vi "FGV_MacroCore.vi"(6 "Final Index":i32, 7 "MacroFGV_Commands":T1, 8 "Error In":errorcluster, 9 "Length":i32, 10 "Start Index":i32, 11 "Macro Command or Info (String)":string) -> (0 "Error Out":errorcluster, 1 "Info Table Array":string[](array[string]), 2 "File IO Cancelled/Error?":bool, 3 "Macro String Array":string[](array[string]), 5 "Saved Macro Path":path)   [LabVIEW 2012]
doc: "SciScan 1.2 160622\nThis is the main FGV which manages the Macro Data"
uses:
  FGV_MacroCore_Commands.ctl
  MacroFileIO_Commands.ctl
  FGV_Macro Settings to GFG_Command.ctl
  Macro Rule/subVIs/MacroRules_FGV_Commands.ctl
  Custom Controls/Setting File Types.ctl
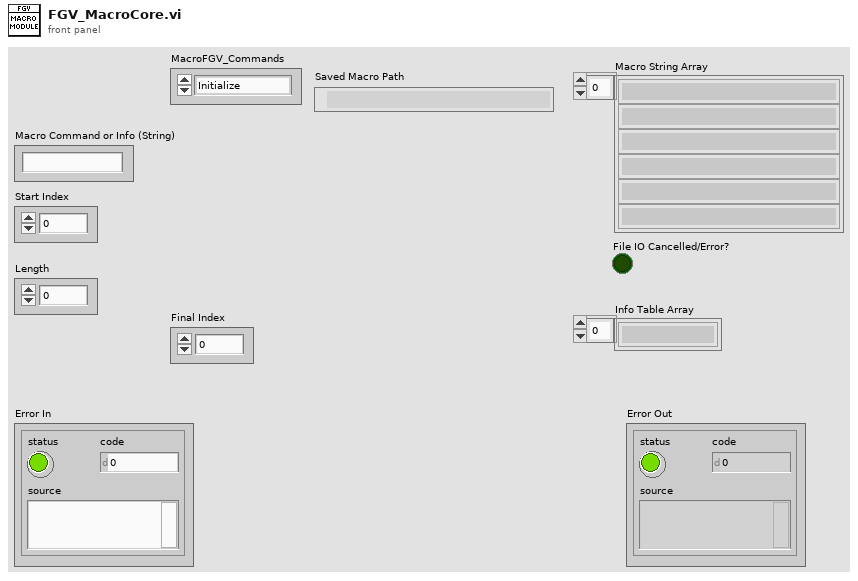
[diagram p1: front panel]
types:
  T1 = typedef "FGV_MacroCore_Commands.ctl" = enum16{"Initialize", "Get Array", "Load macro from file", "Insert Item", "Insert at End", "Edit Parameter String", "Delete instruction", "Move Items", "Save", "SaveAs", "UpdateInfoTable", "Edit Settings File", "New Macro", "Read Temp File", "Delete Multiple"}
  T2 = typedef "MacroFileIO_Commands.ctl" = enum16{"Get Macro Info", "Initialize", "New Macro", "Load Macro", "Save", "Save in today's folder", "Update Settings File", "Add Settings File", "Delete Settings File", "Update Macro Text", "Save As", "Read Temp File"}
  T3 = typedef "MacroRules_FGV_Commands.ctl" = enum16{"Read File", "Get All", "Get Param and Flags"}
  T4 = typedef "FGV_Macro Settings to GFG_Command.ctl" = enum16{"Get Current Settings", "Backup Curent Settings", "Recover Backed up settings", "Overwrite Current Settings"}
  T5 = typedef "Macro_Action_List.ctl" = enum16{"Unknown Command", "2D.Frame.Scan", "2D.Line.Scan", "Load.Settings.File", "Move.To.Position", "Pause", "Z.Stack", "LOOP.Start", "LOOP.End", "Record", "Fast.Z", "Generic", "Slow.Z", "Tiling", "Preset.End"}
  T6 = typedef "Setting File Types.ctl" = enum16{"2D.Frame.Scan.Settings", "2D.Line.Scan.Settings", "Z.Stack.Settings", "HW Settings", "Configuration Settings", "Unknown Settings", "Fast.Z.Settings"}
  T7 = typedef "GFG Variable for IO.ctl" = cluster{"Variable Name":string, "Value (Variant)":variant, "data type":string}
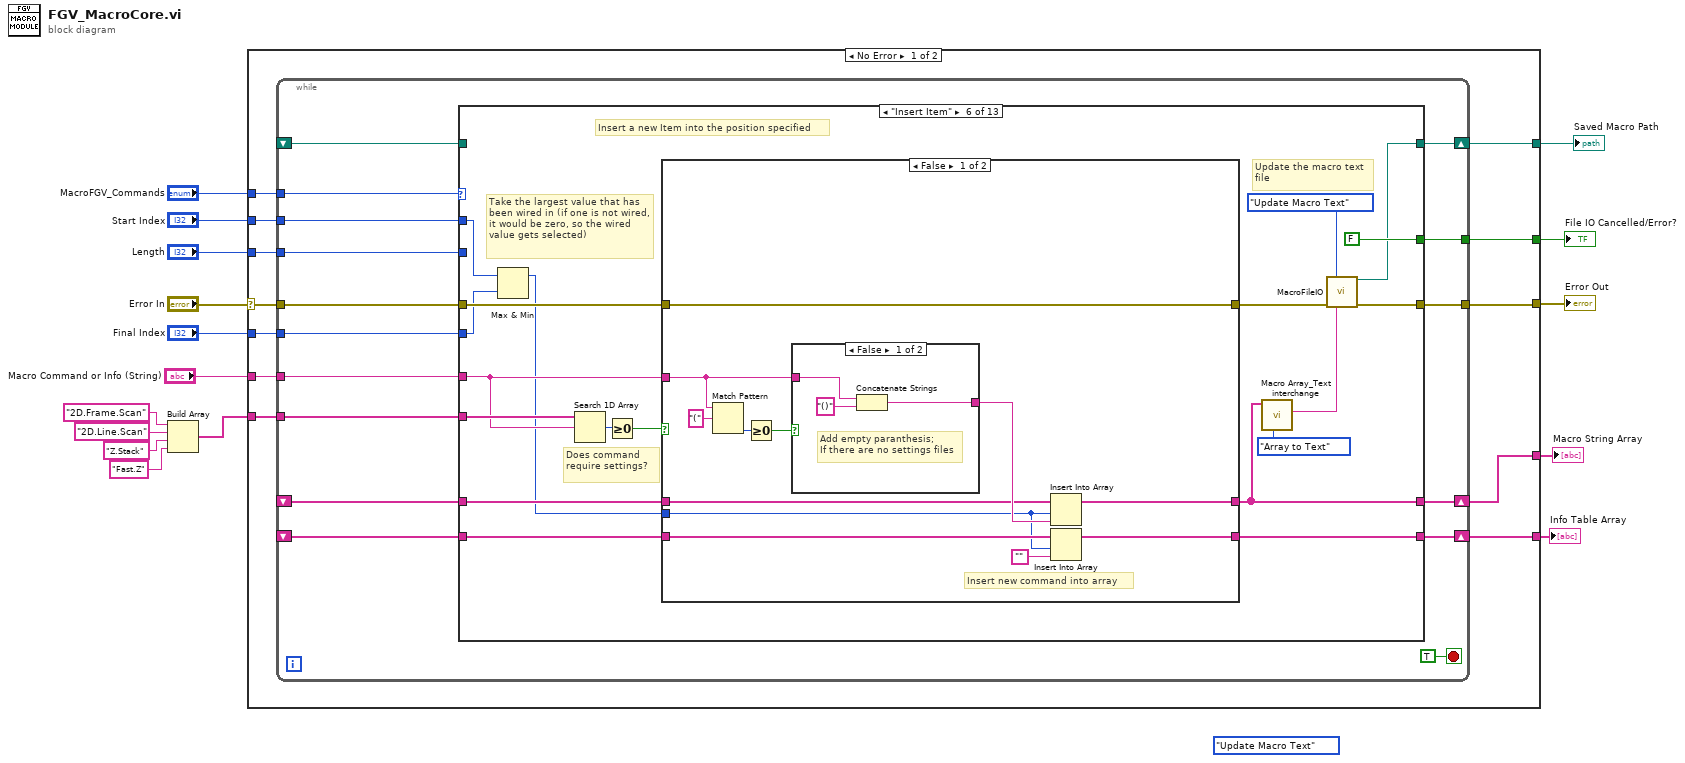
[diagram p0: block diagram]
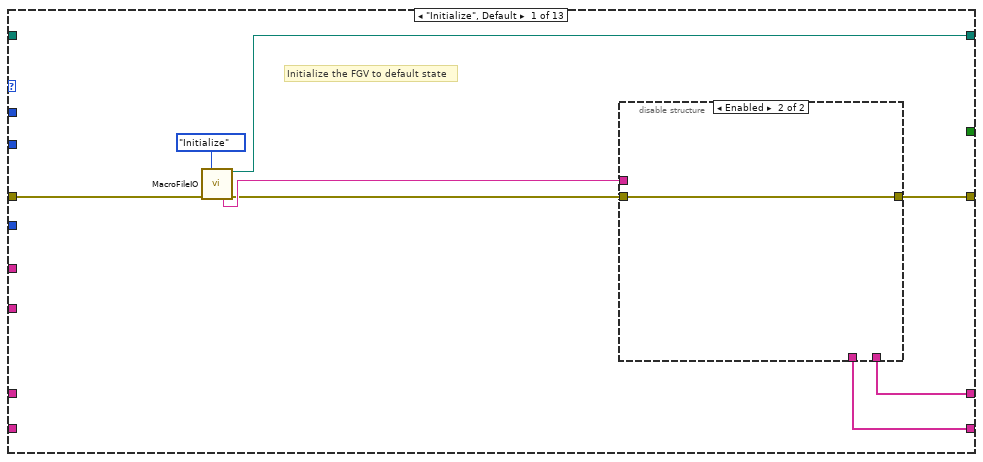
[diagram p2: hidden frame]
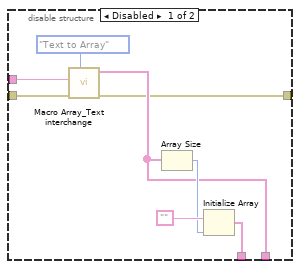
[diagram p3: hidden frame]
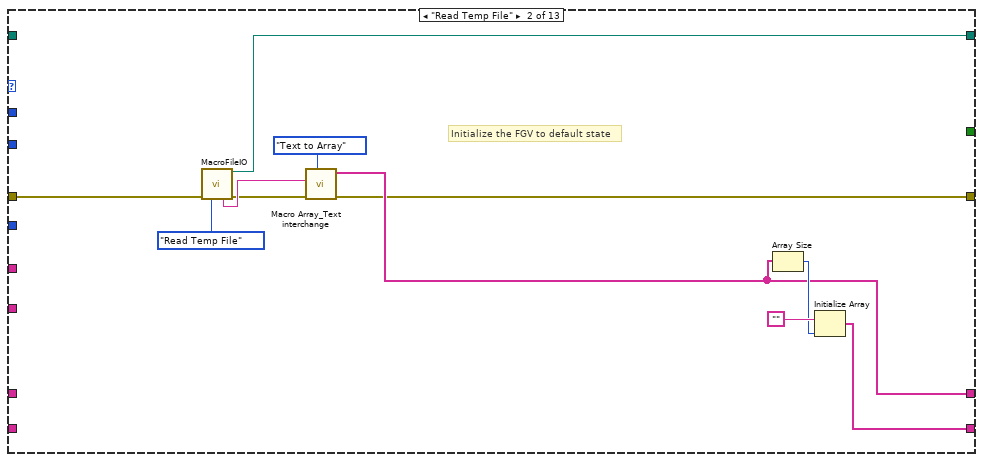
[diagram p4: hidden frame]
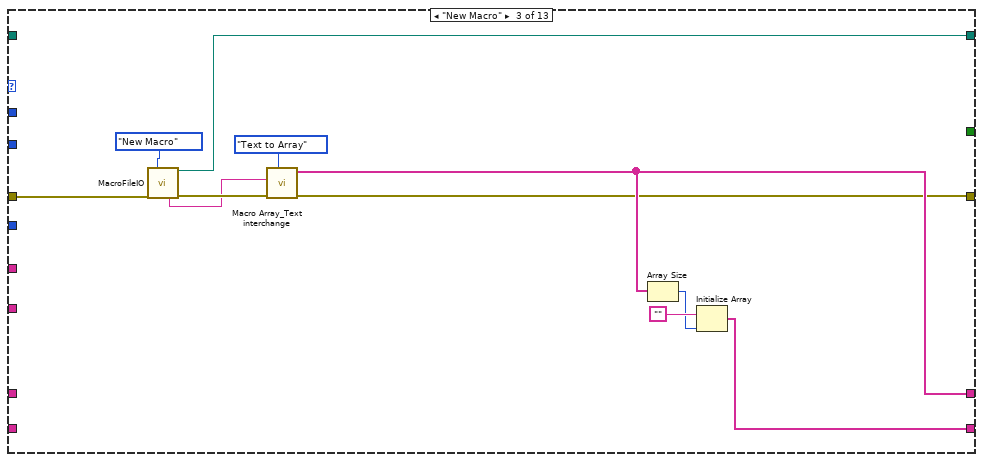
[diagram p5: hidden frame]
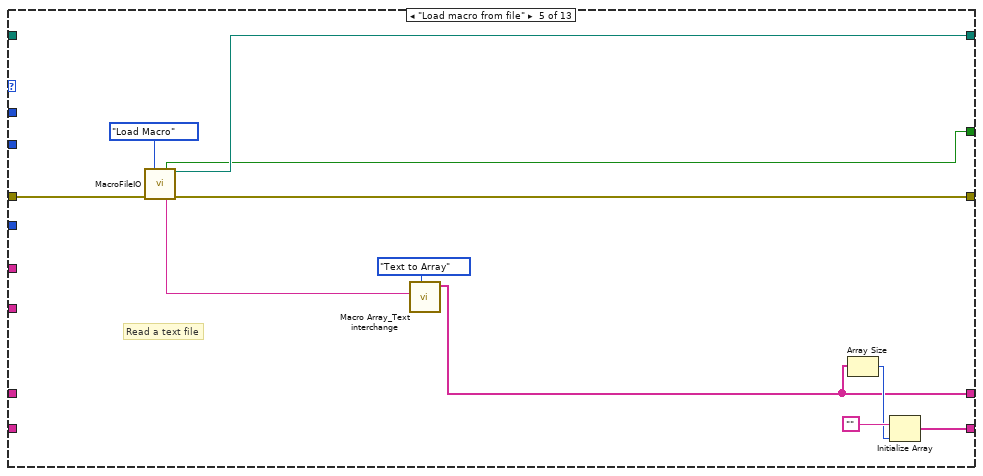
[diagram p7: hidden frame]
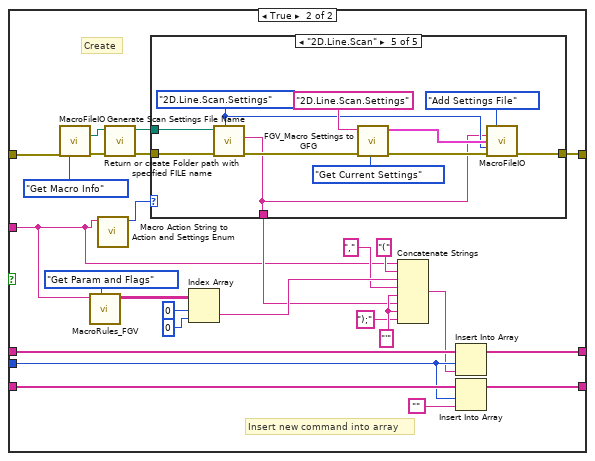
[diagram p9: hidden frame]
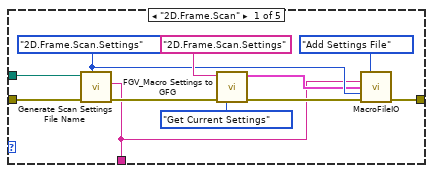
[diagram p10: hidden frame]
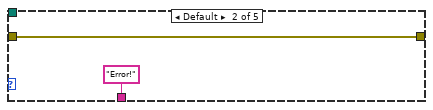
[diagram p11: hidden frame]
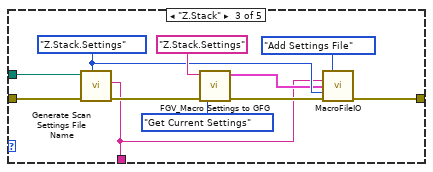
[diagram p12: hidden frame]
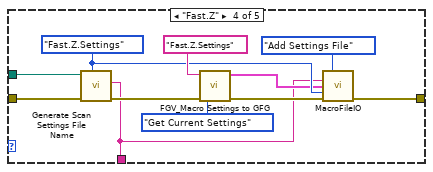
[diagram p13: hidden frame]
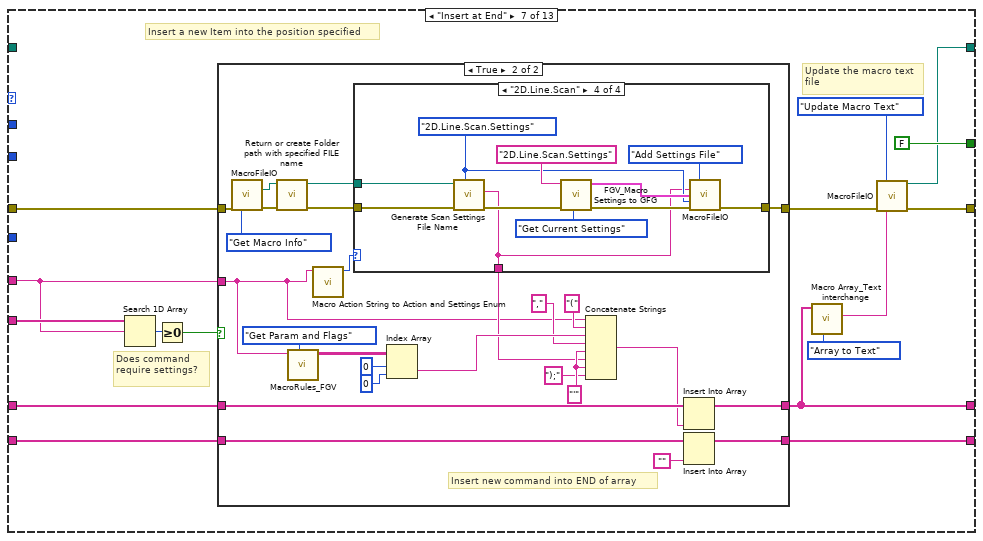
[diagram p14: hidden frame]
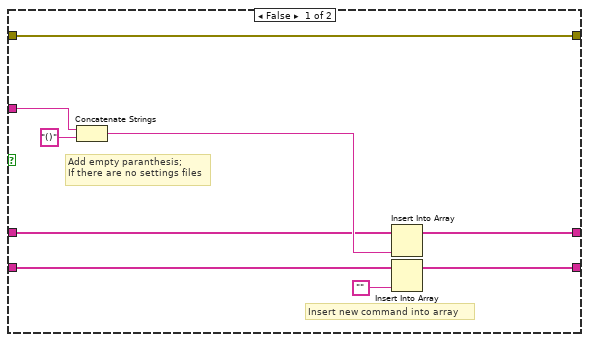
[diagram p15: hidden frame]
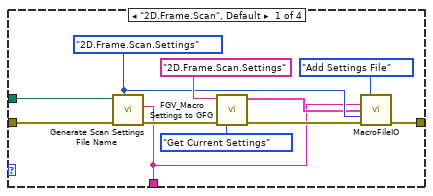
[diagram p16: hidden frame]
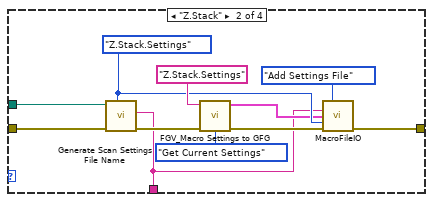
[diagram p17: hidden frame]
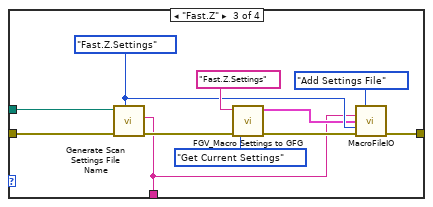
[diagram p18: hidden frame]
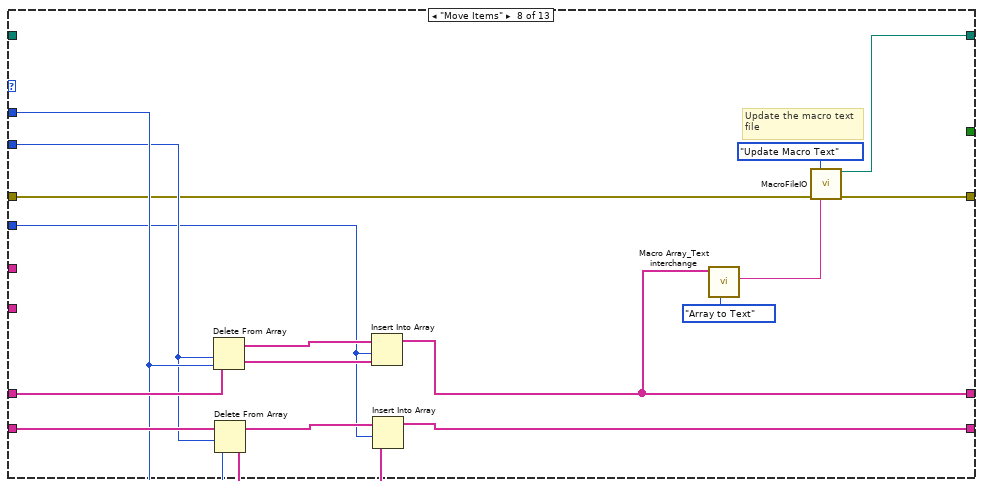
[diagram p19: hidden frame]
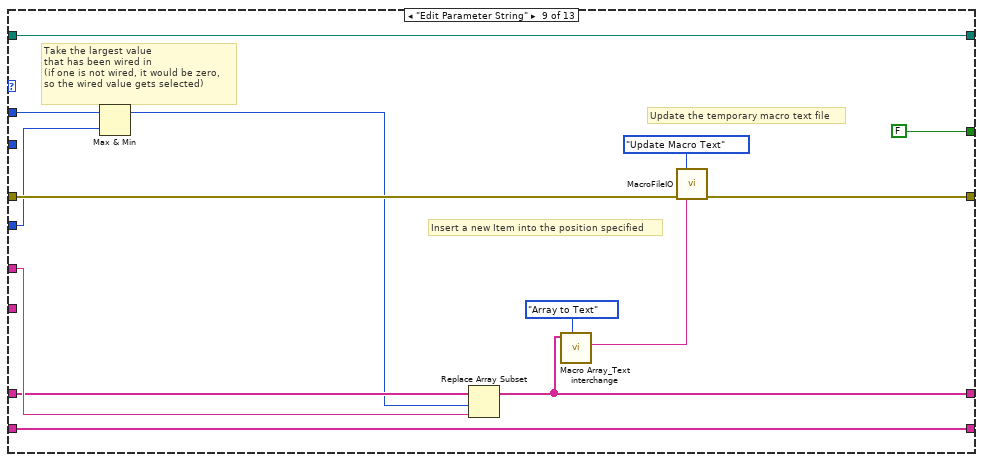
[diagram p20: hidden frame]
diagram:
  (unwired) MacroFileIO_Commands."Update Macro Text" ("MacroFileIO_Command")
  n1 = Build Array("2D.Frame.Scan" ("regular expression"), "2D.Line.Scan" ("regular expression"), "Z.Stack" ("regular expression"), "Fast.Z" ("regular expression")) -> (w3:string[])
  n2 = case shown="No Error" "Error In" {
    selector: "Error In" -> [w27 w463]
    tunnel: "MacroFGV_Commands" -> [w28 _]
    tunnel: "Final Index" -> [w26 _]
    tunnel: [w25 _] -> w13
    tunnel: [w24 w463] -> w12
    tunnel: "Start Index" -> [w23 _]
    tunnel: "Length" -> [w22 _]
    tunnel: [w21 _] -> w9
    tunnel: "Macro Command or Info (String)" -> [w20 _]
    tunnel: [w19 _] -> w7
    tunnel: w3 -> [w18 _]
    tunnel: [w17 _] -> w2
    frame No Error {
      n3 = while {
        tunnel: w28 -> [w43]
        shift-right: [w42] -> w17
        shift-left: _ -> [w41]
        tunnel: w27 -> [w40]
        tunnel: w26 -> [w39]
        tunnel: [w38] -> w25
        tunnel: [w37] -> w24
        tunnel: w23 -> [w36]
        tunnel: w22 -> [w35]
        shift-right: [w34] -> w21
        shift-left: _ -> [w33]
        tunnel: w20 -> [w32]
        shift-right: [w31] -> w19
        shift-left: _ -> [w30]
        tunnel: w18 -> [w29]
        stop <- TRUE stop-if-true
        n4 = case shown="\"Insert Item\"" w43 {
          tunnel: [w50 w70 w81 w87 w92 w102 w206 w303 w330 w339 w369 w420 w450] -> w42
          tunnel: w41 -> [_ _ _ w87 _ _ _ _ w330 _ _ w420 w450]
          tunnel: w40 -> [w51 w71 w82 w86 w94 w110 w214 w302 w322 w338 w378 w419 w447]
          tunnel: w39 -> [_ _ _ _ _ w100 _ w307 w318 w333 _ w413 w423]
          tunnel: [_ _ _ _ w88 FALSE FALSE _ FALSE _ _ _ _] -> w38
          tunnel: [w45 w62 w73 w86 w95 w107 w211 w301 w320 w341 w366 w419 w438] -> w37
          tunnel: w36 -> [_ _ _ _ _ w101 _ w310 w319 w332 w377 w414 w422]
          tunnel: w35 -> [_ _ _ _ _ _ _ w309 _ _ w376 _ _]
          tunnel: [w46 w63 w75 w85 w90 w104 w208 w300 w323 w342 w370 w418 w427] -> w34
          tunnel: w33 -> [_ _ _ w85 _ w112 w216 w316 w327 w359 w381 w418 w428]
          tunnel: w32 -> [_ _ _ _ _ w115 w219 _ w328 _ _ w416 _]
          tunnel: [w47 w64 w74 w84 w96 w109 w213 w308 w326 w356 w379 w415 w449] -> w31
          tunnel: w30 -> [_ _ _ w84 _ w111 w215 w311 w326 w357 w380 w417 w449]
          tunnel: w29 -> [_ _ _ _ _ w116 w220 _ _ _ _ _ _]
          frame "Initialize", Default {
            # "Initialize the FGV to default state"
            n5 = call "MacroFileIO.vi"("MacroFileIO_Command"=MacroFileIO_Commands."Initialize", "Error In"=w51) -> ("Macro File Path OUT"=w50:path, "Macro Text OUT"=w49:string, "Error Out"=w48:errorcluster)  [unwired: 8 in, 3 out]
            n6 = disable-structure shown="Enabled" {
              disable-tunnel: w49 -> [w57 _]
              disable-tunnel: w48 -> [w56 w61]
              disable-tunnel: [w55 _] -> w47
              disable-tunnel: [w54 _] -> w46
              disable-tunnel: [w53 w61] -> w45
              frame Disabled {
                n7 = call "Macro Array_Text interchange.vi"("Command"=enum16{"Array to Text", "Text to Array"}."Text to Array", "error in (no error)"=w56, "Macro Text IN"=w57) -> ("error out"=w53:errorcluster, "Macro Array OUT"=w54:string[])  [unwired: 6 in, 1 out]
                n8 = Array Size(array=w54) -> (size(s)=w59:i32)
                n9 = Initialize Array("", w59) -> (w55:string[])
              }
              frame Enabled {
              }
            }
          }
          frame "Read Temp File" {
            # "Initialize the FGV to default state"
            n10 = call "MacroFileIO.vi"("MacroFileIO_Command"=MacroFileIO_Commands."Read Temp File", "Error In"=w71) -> ("Macro File Path OUT"=w70:path, "Macro Text OUT"=w66:string, "Error Out"=w65:errorcluster)  [unwired: 8 in, 3 out]
            n11 = call "Macro Array_Text interchange.vi"("Command"=enum16{"Array to Text", "Text to Array"}."Text to Array", "error in (no error)"=w65, "Macro Text IN"=w66) -> ("error out"=w62:errorcluster, "Macro Array OUT"=w63:string[])  [unwired: 6 in, 1 out]
            n12 = Array Size(array=w63) -> (size(s)=w68:i32)
            n13 = Initialize Array("", w68) -> (w64:string[])
          }
          frame "New Macro" {
            n14 = call "MacroFileIO.vi"("MacroFileIO_Command"=MacroFileIO_Commands."New Macro", "Error In"=w82) -> ("Macro File Path OUT"=w81:path, "Macro Text OUT"=w76:string, "Error Out"=w77:errorcluster)  [unwired: 8 in, 3 out]
            n15 = call "Macro Array_Text interchange.vi"("Command"=enum16{"Array to Text", "Text to Array"}."Text to Array", "error in (no error)"=w77, "Macro Text IN"=w76) -> ("error out"=w73:errorcluster, "Macro Array OUT"=w75:string[])  [unwired: 6 in, 1 out]
            n16 = Array Size(array=w75) -> (size(s)=w79:i32)
            n17 = Initialize Array("", w79) -> (w74:string[])
          }
          frame "Get Array" {
            # "Returns an array of all the stored commands"
          }
          frame "Load macro from file" {
            # "Read a text file"
            n18 = call "MacroFileIO.vi"("MacroFileIO_Command"=MacroFileIO_Commands."Load Macro" ("FGV_MacroFileIO_Command"), "Error In"=w94) -> ("File IO Cancelled/NotFound?"=w88:bool, "Macro File Path OUT"=w92:path, "Macro Text OUT"=w91:string, "Error Out"=w95:errorcluster)  [unwired: 8 in, 2 out]
            n19 = call "Macro Array_Text interchange.vi"("Command"=enum16{"Array to Text", "Text to Array"}."Text to Array", "Macro Text IN"=w91) -> ("Macro Array OUT"=w90:string[])  [unwired: 7 in, 2 out]
            n20 = Array Size(array=w90) -> (size(s)=w97:i32)
            n21 = Initialize Array("", w97) -> (w96:string[])
          }
          frame "Insert Item" {
            # "Take the largest value that has been wired in (if one is not wired, it would be zero, so the wired value gets selected)"
            # "Update the macro text\nfile"
            # "Does command require settings?"
            # "Insert a new Item into the position specified"
            n22 = Max & Min(x=w101, y=w100) -> (max(x,y)=w99:i32)  [unwired: 1 out]
            n23 = Search 1D Array(1D array=w116, element=w115) -> (index of element=w114:i32)  [unwired: 1 in]
            n24 = Greater Or Equal To 0?(x=w114) -> (x >= 0?=w113:bool)
            n25 = case shown="False" w113 {
              tunnel: w115 -> [w121 w134]
              tunnel: w112 -> [w127 w151]
              tunnel: w111 -> [w126 w150]
              tunnel: w110 -> [w122 w152]
              tunnel: w99 -> [w125 w148]
              tunnel: [w124 w144] -> w104
              tunnel: [w123 w146] -> w109
              tunnel: [w122 w143] -> w108
              frame False {
                # "Insert new command into array"
                n26 = Match Pattern(string=w121, regular expression="(") -> (offset past match=w119:i32)  [unwired: 1 in, 3 out]
                n27 = Greater Or Equal To 0?(x=w119) -> (x >= 0?=w118:bool)
                n28 = case shown="False" w118 {
                  tunnel: [w131 w133] -> w128
                  tunnel: w121 -> [w130 w133]
                  frame False {
                    # "Add empty paranthesis;\nIf there are no settings files"
                    n29 = Concatenate Strings(w130, "()" ("string")) -> (w131:string)
                  }
                  frame True {
                  }
                }
                n30 = Insert Into Array(array=w127, index=w125, new element=w128) -> (w124:string[])
                n31 = Insert Into Array(array=w126, index=w125, new element="") -> (w123:string[])
              }
              frame True {
                w154 = "'" ("string")
                # "Create"
                # "Insert new command into array"
                n32 = call "MacroFileIO.vi"("MacroFileIO_Command"=MacroFileIO_Commands."Get Macro Info", "Error In"=w152) -> ("Temp File path"=w145:path, "Error Out"=w158:errorcluster)  [unwired: 8 in, 4 out]
                n33 = call "MacroRules_FGV.vi"("MacroRules_FGV_Commands"=MacroRules_FGV_Commands."Get Param and Flags", "Command Name IN"=w134) -> ("Parameters"=w141:string[][])  [unwired: 5 in, 4 out]
                n34 = call "Macro Action String to Action and Settings Enum.vi"("Action String IN"=w134) -> ("Action Enum OUT"=w135:T5)  [unwired: 7 in, 3 out]
                n35 = call "Return or create Folder path with specified FILE name.vi"("error in (no error)"=w158, "File Path IN"=w145) -> ("error out"=w156:errorcluster, "Folder Path OUT"=w157:path)  [unwired: 8 in]
                n36 = case shown="\"2D.Line.Scan\"" w135 {
                  tunnel: w157 -> [w169 _ w182 w193 w205]
                  tunnel: w156 -> [w170 w172 w183 w194 w204]
                  tunnel: [w161 w172 w174 w185 w197] -> w143
                  tunnel: [w160 "Error!" ("New Settings Filename") w173 w184 w195] -> w136
                  frame "2D.Frame.Scan" {
                    w164 = Setting_File_Types."2D.Frame.Scan.Settings" ("Setting File Type")
                    n37 = call "Generate Scan Settings File Name.vi"("Setting File Type"=w164, "error in (no error)"=w170, "Settings Folder Path IN"=w169) -> ("error out"=w166:errorcluster, "New Settings Filename"=w160:string)  [unwired: 6 in, 1 out]
                    n38 = call "FGV_Macro Settings to GFG.vi"("FGV_Macro Settings to GFG_Command"=FGV_Macro_Settings_to_GFG_Command."Get Current Settings", "error in (no error)"=w166, "Settings type string IN"="2D.Frame.Scan.Settings") -> ("error out"=w163:errorcluster, "Current Settings OUT"=w162:T7[])  [unwired: 6 in, 1 out]
                    n39 = call "MacroFileIO.vi"("MacroFileIO_Command"=MacroFileIO_Commands."Add Settings File", "Settings File Name IN"=w160, "Settings Data IN"=w162, "Setting File Type"=w164, "Error In"=w163) -> ("Error Out"=w161:errorcluster)  [unwired: 5 in, 5 out]
                  }
                  frame Default {
                  }
                  frame "Z.Stack" {
                    w176 = Setting_File_Types."Z.Stack.Settings" ("Setting File Type")
                    n40 = call "Generate Scan Settings File Name.vi"("Setting File Type"=w176, "error in (no error)"=w183, "Settings Folder Path IN"=w182) -> ("error out"=w179:errorcluster, "New Settings Filename"=w173:string)  [unwired: 6 in, 1 out]
                    n41 = call "FGV_Macro Settings to GFG.vi"("FGV_Macro Settings to GFG_Command"=FGV_Macro_Settings_to_GFG_Command."Get Current Settings", "error in (no error)"=w179, "Settings type string IN"="Z.Stack.Settings") -> ("error out"=w177:errorcluster, "Current Settings OUT"=w175:T7[])  [unwired: 6 in, 1 out]
                    n42 = call "MacroFileIO.vi"("MacroFileIO_Command"=MacroFileIO_Commands."Add Settings File", "Settings File Name IN"=w173, "Settings Data IN"=w175, "Setting File Type"=w176, "Error In"=w177) -> ("Error Out"=w174:errorcluster)  [unwired: 5 in, 5 out]
                  }
                  frame "Fast.Z" {
                    w187 = Setting_File_Types."Fast.Z.Settings" ("Setting File Type")
                    n43 = call "Generate Scan Settings File Name.vi"("Setting File Type"=w187, "error in (no error)"=w194, "Settings Folder Path IN"=w193) -> ("error out"=w190:errorcluster, "New Settings Filename"=w184:string)  [unwired: 6 in, 1 out]
                    n44 = call "FGV_Macro Settings to GFG.vi"("FGV_Macro Settings to GFG_Command"=FGV_Macro_Settings_to_GFG_Command."Get Current Settings", "error in (no error)"=w190, "Settings type string IN"="Fast.Z.Settings") -> ("error out"=w188:errorcluster, "Current Settings OUT"=w186:T7[])  [unwired: 6 in, 1 out]
                    n45 = call "MacroFileIO.vi"("MacroFileIO_Command"=MacroFileIO_Commands."Add Settings File", "Settings File Name IN"=w184, "Settings Data IN"=w186, "Setting File Type"=w187, "Error In"=w188) -> ("Error Out"=w185:errorcluster)  [unwired: 5 in, 5 out]
                  }
                  frame "2D.Line.Scan" {
                    w196 = Setting_File_Types."2D.Line.Scan.Settings" ("Setting File Type")
                    n46 = call "Generate Scan Settings File Name.vi"("Setting File Type"=w196, "error in (no error)"=w204, "Settings Folder Path IN"=w205) -> ("error out"=w201:errorcluster, "New Settings Filename"=w195:string)  [unwired: 6 in, 1 out]
                    n47 = call "FGV_Macro Settings to GFG.vi"("FGV_Macro Settings to GFG_Command"=FGV_Macro_Settings_to_GFG_Command."Get Current Settings", "error in (no error)"=w201, "Settings type string IN"="2D.Line.Scan.Settings") -> ("error out"=w198:errorcluster, "Current Settings OUT"=w199:T7[])  [unwired: 6 in, 1 out]
                    n48 = call "MacroFileIO.vi"("MacroFileIO_Command"=MacroFileIO_Commands."Add Settings File", "Settings File Name IN"=w195, "Settings Data IN"=w199, "Setting File Type"=w196, "Error In"=w198) -> ("Error Out"=w197:errorcluster)  [unwired: 5 in, 5 out]
                  }
                }
                n49 = Index Array(array=w141, index (row)=0, index (col)=0 ("disabled index (col)")) -> (element=w138:string)
                n50 = Concatenate Strings(w134, "(" ("string"), w138, "," ("string"), w154, w136, w154, ");" ("string")) -> (w147:string)
                n51 = Insert Into Array(array=w151, index=w148, new element=w147) -> (w144:string[])
                n52 = Insert Into Array(array=w150, index=w148, new element="") -> (w146:string[])
              }
            }
            n53 = call "Macro Array_Text interchange.vi"("Command"=enum16{"Array to Text", "Text to Array"}."Array to Text", "Macro Array IN"=w104) -> ("Macro Text OUT"=w103:string)  [unwired: 7 in, 2 out]
            n54 = call "MacroFileIO.vi"("MacroFileIO_Command"=MacroFileIO_Commands."Update Macro Text", "Error In"=w108, "Macro Text IN"=w103) -> ("Macro File Path OUT"=w102:path, "Error Out"=w107:errorcluster)  [unwired: 7 in, 4 out]
          }
          frame "Insert at End" {
            # "Update the macro text\nfile"
            # "Does command require settings?"
            # "Insert a new Item into the position specified"
            n55 = Search 1D Array(1D array=w220, element=w219) -> (index of element=w218:i32)  [unwired: 1 in]
            n56 = Greater Or Equal To 0?(x=w218) -> (x >= 0?=w217:bool)
            n57 = case shown="True" w217 {
              tunnel: w219 -> [w229 w232]
              tunnel: w216 -> [w226 w250]
              tunnel: w215 -> [w225 w249]
              tunnel: w214 -> [w222 w251]
              tunnel: [w224 w245] -> w208
              tunnel: [w223 w247] -> w213
              tunnel: [w222 w244] -> w212
              frame False {
                # "Add empty paranthesis;\nIf there are no settings files"
                # "Insert new command into array"
                n58 = Concatenate Strings(w229, "()" ("string")) -> (w227:string)
                n59 = Insert Into Array(array=w226, new element=w227) -> (w224:string[])  [unwired: 1 in]
                n60 = Insert Into Array(array=w225, new element="") -> (w223:string[])  [unwired: 1 in]
              }
              frame True {
                w242 = "'" ("string")
                # "Insert new command into END of array"
                n61 = call "MacroFileIO.vi"("MacroFileIO_Command"=MacroFileIO_Commands."Get Macro Info", "Error In"=w251) -> ("Temp File path"=w246:path, "Error Out"=w254:errorcluster)  [unwired: 8 in, 4 out]
                n62 = call "Return or create Folder path with specified FILE name.vi"("error in (no error)"=w254, "File Path IN"=w246) -> ("error out"=w252:errorcluster, "Folder Path OUT"=w253:path)  [unwired: 8 in]
                n63 = call "MacroRules_FGV.vi"("MacroRules_FGV_Commands"=MacroRules_FGV_Commands."Get Param and Flags", "Command Name IN"=w232) -> ("Parameters"=w239:string[][])  [unwired: 5 in, 4 out]
                n64 = call "Macro Action String to Action and Settings Enum.vi"("Action String IN"=w232) -> ("Action Enum OUT"=w231:T5)  [unwired: 7 in, 3 out]
                n65 = case shown="\"2D.Line.Scan\"" w231 {
                  tunnel: w253 -> [w265 w276 w287 w299]
                  tunnel: w252 -> [w266 w277 w288 w298]
                  tunnel: [w257 w268 w279 w291] -> w244
                  tunnel: [w256 w267 w278 w289] -> w234
                  frame "2D.Frame.Scan", Default {
                    w260 = Setting_File_Types."2D.Frame.Scan.Settings" ("Setting File Type")
                    n66 = call "Generate Scan Settings File Name.vi"("Setting File Type"=w260, "error in (no error)"=w266, "Settings Folder Path IN"=w265) -> ("error out"=w262:errorcluster, "New Settings Filename"=w256:string)  [unwired: 6 in, 1 out]
                    n67 = call "FGV_Macro Settings to GFG.vi"("FGV_Macro Settings to GFG_Command"=FGV_Macro_Settings_to_GFG_Command."Get Current Settings", "error in (no error)"=w262, "Settings type string IN"="2D.Frame.Scan.Settings") -> ("error out"=w259:errorcluster, "Current Settings OUT"=w258:T7[])  [unwired: 6 in, 1 out]
                    n68 = call "MacroFileIO.vi"("MacroFileIO_Command"=MacroFileIO_Commands."Add Settings File", "Settings File Name IN"=w256, "Settings Data IN"=w258, "Setting File Type"=w260, "Error In"=w259) -> ("Error Out"=w257:errorcluster)  [unwired: 5 in, 5 out]
                  }
                  frame "Z.Stack" {
                    w270 = Setting_File_Types."Z.Stack.Settings" ("Setting File Type")
                    n69 = call "Generate Scan Settings File Name.vi"("Setting File Type"=w270, "error in (no error)"=w277, "Settings Folder Path IN"=w276) -> ("error out"=w273:errorcluster, "New Settings Filename"=w267:string)  [unwired: 6 in, 1 out]
                    n70 = call "FGV_Macro Settings to GFG.vi"("FGV_Macro Settings to GFG_Command"=FGV_Macro_Settings_to_GFG_Command."Get Current Settings", "error in (no error)"=w273, "Settings type string IN"="Z.Stack.Settings") -> ("error out"=w271:errorcluster, "Current Settings OUT"=w269:T7[])  [unwired: 6 in, 1 out]
                    n71 = call "MacroFileIO.vi"("MacroFileIO_Command"=MacroFileIO_Commands."Add Settings File", "Settings File Name IN"=w267, "Settings Data IN"=w269, "Setting File Type"=w270, "Error In"=w271) -> ("Error Out"=w268:errorcluster)  [unwired: 5 in, 5 out]
                  }
                  frame "Fast.Z" {
                    w281 = Setting_File_Types."Fast.Z.Settings" ("Setting File Type")
                    n72 = call "Generate Scan Settings File Name.vi"("Setting File Type"=w281, "error in (no error)"=w288, "Settings Folder Path IN"=w287) -> ("error out"=w284:errorcluster, "New Settings Filename"=w278:string)  [unwired: 6 in, 1 out]
                    n73 = call "FGV_Macro Settings to GFG.vi"("FGV_Macro Settings to GFG_Command"=FGV_Macro_Settings_to_GFG_Command."Get Current Settings", "error in (no error)"=w284, "Settings type string IN"="Fast.Z.Settings") -> ("error out"=w282:errorcluster, "Current Settings OUT"=w280:T7[])  [unwired: 6 in, 1 out]
                    n74 = call "MacroFileIO.vi"("MacroFileIO_Command"=MacroFileIO_Commands."Add Settings File", "Settings File Name IN"=w278, "Settings Data IN"=w280, "Setting File Type"=w281, "Error In"=w282) -> ("Error Out"=w279:errorcluster)  [unwired: 5 in, 5 out]
                  }
                  frame "2D.Line.Scan" {
                    w290 = Setting_File_Types."2D.Line.Scan.Settings" ("Setting File Type")
                    n75 = call "Generate Scan Settings File Name.vi"("Setting File Type"=w290, "error in (no error)"=w298, "Settings Folder Path IN"=w299) -> ("error out"=w295:errorcluster, "New Settings Filename"=w289:string)  [unwired: 6 in, 1 out]
                    n76 = call "FGV_Macro Settings to GFG.vi"("FGV_Macro Settings to GFG_Command"=FGV_Macro_Settings_to_GFG_Command."Get Current Settings", "error in (no error)"=w295, "Settings type string IN"="2D.Line.Scan.Settings") -> ("error out"=w292:errorcluster, "Current Settings OUT"=w293:T7[])  [unwired: 6 in, 1 out]
                    n77 = call "MacroFileIO.vi"("MacroFileIO_Command"=MacroFileIO_Commands."Add Settings File", "Settings File Name IN"=w289, "Settings Data IN"=w293, "Setting File Type"=w290, "Error In"=w292) -> ("Error Out"=w291:errorcluster)  [unwired: 5 in, 5 out]
                  }
                }
                n78 = Index Array(array=w239, index (row)=0, index (col)=0 ("disabled index (col)")) -> (element=w236:string)
                n79 = Concatenate Strings(w232, "(" ("string"), w236, "," ("string"), w242, w234, w242, ");" ("string")) -> (w233:string)
                n80 = Insert Into Array(array=w250, new element=w233) -> (w245:string[])  [unwired: 1 in]
                n81 = Insert Into Array(array=w249, new element="") -> (w247:string[])  [unwired: 1 in]
              }
            }
            n82 = call "Macro Array_Text interchange.vi"("Command"=enum16{"Array to Text", "Text to Array"}."Array to Text", "Macro Array IN"=w208) -> ("Macro Text OUT"=w207:string)  [unwired: 7 in, 2 out]
            n83 = call "MacroFileIO.vi"("MacroFileIO_Command"=MacroFileIO_Commands."Update Macro Text", "Error In"=w212, "Macro Text IN"=w207) -> ("Macro File Path OUT"=w206:path, "Error Out"=w211:errorcluster)  [unwired: 7 in, 4 out]
          }
          frame "Move Items" {
            # "Update the macro text\nfile"
            n84 = Delete From Array(array=w316, length=w309, index=w310) -> (deleted portion=w314:string[], array with subset deleted=w315:string[])
            n85 = Delete From Array(array=w311, length=w309, index=w310) -> (deleted portion=w313:string[], array with subset deleted=w312:string[])
            n86 = Insert Into Array(array=w315, index=w307, new element=w314) -> (w300:string[])
            n87 = Insert Into Array(array=w312, index=w307, new element=w313) -> (w308:string[])
            n88 = call "Macro Array_Text interchange.vi"("Command"=enum16{"Array to Text", "Text to Array"}."Array to Text", "Macro Array IN"=w300) -> ("Macro Text OUT"=w304:string)  [unwired: 7 in, 2 out]
            n89 = call "MacroFileIO.vi"("MacroFileIO_Command"=MacroFileIO_Commands."Update Macro Text", "Error In"=w302, "Macro Text IN"=w304) -> ("Macro File Path OUT"=w303:path, "Error Out"=w301:errorcluster)  [unwired: 7 in, 4 out]
          }
          frame "Edit Parameter String" {
            # "Take the largest value\nthat has been wired in\n(if one is not wired, it would be zero,\nso the wired value gets selected)"
            # "Update the temporary macro text file"
            # "Insert a new Item into the position specified"
            n90 = Max & Min(x=w319, y=w318) -> (max(x,y)=w317:i32)  [unwired: 1 out]
            n91 = Replace Array Subset(array=w327, new element=w328, index=w317) -> (w323:string[])
            n92 = call "Macro Array_Text interchange.vi"("Command"=enum16{"Array to Text", "Text to Array"}."Array to Text", "Macro Array IN"=w323) -> ("Macro Text OUT"=w325:string)  [unwired: 7 in, 2 out]
            n93 = call "MacroFileIO.vi"("MacroFileIO_Command"=MacroFileIO_Commands."Update Macro Text", "Error In"=w322, "Macro Text IN"=w325) -> ("Error Out"=w320:errorcluster)  [unwired: 7 in, 5 out]
          }
          frame "Delete instruction" {
            # "Take the largest value that has been wired in (if one is not wired, it would be zero, so the wired value gets selected)"
            # "Delete Settings file ony if there is a valid setup file name:\n(i.e., the command should require a settings file)"
            # "Remove any apostrophe"
            # "Update the macro text\nfile"
            # "Delete a command from  the array at the specified Index"
            n94 = Max & Min(x=w332, y=w333) -> (max(x,y)=w331:i32)  [unwired: 1 out]
            n95 = call "MacroFileIO.vi"("MacroFileIO_Command"=MacroFileIO_Commands."Get Macro Info", "Error In"=w338) -> ("Error Out"=w334:errorcluster)  [unwired: 8 in, 5 out]
            n96 = Delete From Array(array=w359, length=1, index=w331) -> (deleted portion=w355:string[], array with subset deleted=w342:string[])
            n97 = Delete From Array(array=w357, length=1, index=w331) -> (array with subset deleted=w356:string[])  [unwired: 1 out]
            n98 = Index Array(array=w355, index=0) -> (element=w353:string)
            n99 = call "Decompose Command String.vi"("Command IN"=w353) -> ("Parameter Table"=w352:string[][])  [unwired: 7 in, 3 out]
            n100 = Index Array(array=w352, index (row)=0, index (col)=1 ("disabled index (col)")) -> (element=w349:string)
            n101 = Search and Replace String(replace all?=TRUE ("replace all? (F)"), input string=w349, search string="'", error in=w334) -> (result string=w340:string, error out=w336:errorcluster)  [unwired: 4 in, 2 out]
            n102 = Empty String/Path?(string/path=w340) -> (empty?=w335:bool)
            n103 = case shown="False" w335 {
              tunnel: w336 -> [w364 w365]
              tunnel: [w362 w365] -> w343
              tunnel: w340 -> [w361 _]
              frame False {
                n104 = call "MacroFileIO.vi"("MacroFileIO_Command"=MacroFileIO_Commands."Delete Settings File", "Settings File Name IN"=w361, "Error In"=w364) -> ("Error Out"=w362:errorcluster)  [unwired: 7 in, 5 out]
              }
              frame True {
              }
            }
            n105 = call "Macro Array_Text interchange.vi"("Command"=enum16{"Array to Text", "Text to Array"}."Array to Text", "Macro Array IN"=w342) -> ("Macro Text OUT"=w344:string)  [unwired: 7 in, 2 out]
            n106 = call "MacroFileIO.vi"("MacroFileIO_Command"=MacroFileIO_Commands."Update Macro Text", "Error In"=w343, "Macro Text IN"=w344) -> ("Macro File Path OUT"=w339:path, "Error Out"=w341:errorcluster)  [unwired: 7 in, 4 out]
          }
          frame "Delete Multiple" {
            # "Update the macro text\nfile"
            # "Start deleting from LAST element and work upwards"
            # "Delete a Block of commands from  the array specified bys START INDEX and LENGTH"
            n107 = Decrement(x=w376) -> (x-1=w375:i32)
            n108 = Add(x=w377, y=w375) -> (x+y=w374:i32)
            n109 = for {
              N: w376 -> [_]
              tunnel: w381 -> [w405]
              tunnel: w380 -> [w403]
              tunnel: [w402] -> w379
              tunnel: [w392] -> w370
              tunnel: [w382] -> w368
              tunnel: w378 -> [w390]
              tunnel: w377 -> [_]
              tunnel: w374 -> [w385]
              i -> [w384]
              # "Delete Settings file ony if there is a valid setup file name (i.e., the command should require a settings file)"
              # "Remove any apostrophe"
              n110 = Subtract(x=w385, y=w384) -> (x-y=w383:i32)
              n111 = call "MacroFileIO.vi"("MacroFileIO_Command"=MacroFileIO_Commands."Get Macro Info", "Error In"=w390) -> ("Error Out"=w386:errorcluster)  [unwired: 8 in, 5 out]
              n112 = Delete From Array(array=w405, length=1, index=w383) -> (deleted portion=w401:string[], array with subset deleted=w392:string[])
              n113 = Delete From Array(array=w403, length=1, index=w383) -> (array with subset deleted=w402:string[])  [unwired: 1 out]
              n114 = Index Array(array=w401, index=0) -> (element=w399:string)
              n115 = call "Decompose Command String.vi"("Command IN"=w399) -> ("Parameter Table"=w398:string[][])  [unwired: 7 in, 3 out]
              n116 = Index Array(array=w398, index (row)=0, index (col)=1 ("disabled index (col)")) -> (element=w395:string)
              n117 = Search and Replace String(replace all?=TRUE ("replace all? (F)"), input string=w395, search string="'", error in=w386) -> (result string=w391:string, error out=w388:errorcluster)  [unwired: 4 in, 2 out]
              n118 = Empty String/Path?(string/path=w391) -> (empty?=w387:bool)
              n119 = case shown="False" w387 {
                tunnel: w388 -> [w410 w411]
                tunnel: [w408 w411] -> w382
                tunnel: w391 -> [w407 _]
                frame False {
                  n120 = call "MacroFileIO.vi"("MacroFileIO_Command"=MacroFileIO_Commands."Delete Settings File", "Settings File Name IN"=w407, "Error In"=w410) -> ("Error Out"=w408:errorcluster)  [unwired: 7 in, 5 out]
                }
                frame True {
                }
              }
            }
            n121 = call "Macro Array_Text interchange.vi"("Command"=enum16{"Array to Text", "Text to Array"}."Array to Text", "error in (no error)"=w368, "Macro Array IN"=w370) -> ("error out"=w367:errorcluster, "Macro Text OUT"=w371:string)  [unwired: 6 in, 1 out]
            n122 = call "MacroFileIO.vi"("MacroFileIO_Command"=MacroFileIO_Commands."Update Macro Text", "Error In"=w367, "Macro Text IN"=w371) -> ("Macro File Path OUT"=w369:path, "Error Out"=w366:errorcluster)  [unwired: 7 in, 4 out]
          }
          frame "UpdateInfoTable" {
            # "Take the largest value\nthat has been wired in\n(if one is not wired, it would be zero,\nso the wired value gets selected)"
            # "This case inserts an information into the 'Macro Information Table' at the position specified"
            n123 = Max & Min(x=w414, y=w413) -> (max(x,y)=w412:i32)  [unwired: 1 out]
            n124 = Replace Array Subset(array=w417, new element=w416, index=w412) -> (w415:string[])
          }
          frame "Edit Settings File" {
            w435 = 0 ("index (row)")
            # "Take the largest value that has been wired in (if one is not wired, it would be zero, so the wired value gets selected)"
            # "Check if argument name is wrong; correct it\nif it is."
            n125 = Max & Min(x=w422, y=w423) -> (max(x,y)=w421:i32)  [unwired: 1 out]
            n126 = Index Array(array=w428, index=w421) -> (element=w446:string)
            n127 = call "Decompose Command String.vi"("Error In"=w447, "Command IN"=w446) -> ("Error Out"=w443:errorcluster, "Parameter Table"=w445:string[][], "Action"=w424:string)  [unwired: 6 in, 1 out]
            n128 = call "MacroRules_FGV.vi"("MacroRules_FGV_Commands"=MacroRules_FGV_Commands."Get Param and Flags", "Command Name IN"=w424) -> ("Parameters"=w433:string[][])  [unwired: 5 in, 4 out]
            n129 = Index Array(array=w445, index (row) #1=w435, index (col) #1=1 ("disabled index (col)"), index (row) #2=w435, index (col) #2=w435) -> (element #1=w425:string, element #2=w430:string)
            n130 = Index Array(array=w433, index (row)=0, index (col)=0 ("disabled index (col)")) -> (element=w426:string)
            n131 = Equal?(x=w430, y=w426) -> (x = y?=w429:bool)
            n132 = case shown="False" w429 {
              tunnel: w428 -> [w455 w462]
              tunnel: [w454 w462] -> w427
              tunnel: w426 -> [w457 _]
              tunnel: w425 -> [w456 _]
              tunnel: w421 -> [w453 _]
              tunnel: w424 -> [w452 _]
              frame False {
                w460 = "'" ("string")
                n133 = Concatenate Strings(w452, "(" ("string"), w457, "," ("string"), w460, w456, w460, ");" ("string")) -> (w451:string)
                n134 = Replace Array Subset(array=w455, new element=w451, index=w453) -> (w454:string[])
              }
              frame True {
              }
            }
            n135 = call "Macro Action String to Action and Settings Enum.vi"("error in (no error)"=w443, "Action String IN"=w424) -> ("error out"=w436:errorcluster, "Settings File Type OUT (String)"=w437:string, "Setting File Type OUT"=w442:T6)  [unwired: 6 in, 1 out]
            n136 = call "FGV_Macro Settings to GFG.vi"("FGV_Macro Settings to GFG_Command"=FGV_Macro_Settings_to_GFG_Command."Get Current Settings", "error in (no error)"=w436, "Settings type string IN"=w437) -> ("error out"=w439:errorcluster, "Current Settings OUT"=w440:T7[])  [unwired: 6 in, 1 out]
            n137 = call "MacroFileIO.vi"("MacroFileIO_Command"=MacroFileIO_Commands."Update Settings File", "Settings File Name IN"=w425, "Settings Data IN"=w440, "Setting File Type"=w442, "Error In"=w439) -> ("Error Out"=w438:errorcluster)  [unwired: 5 in, 5 out]
          }
        }
      }
    }
    frame Error {
    }
  }
  "Error Out" <- w12
  "File IO Cancelled/Error?" <- w13
  "Macro String Array" <- w9
  "Info Table Array" <- w7
  "Saved Macro Path" <- w2
